vi "Debug C API.vi"() -> ()   [LabVIEW 2023]
doc: "Example to verify functionality using cAPIs"
panel:
  in  "CAPI Path":path
  in  "Output channel name":string[](array[string])=["Connector0_DIOPORT2", "Connector0_DIOPORT3", "Connector1_DIOPORT2", "Connector1_DIOPORT3"]
  in  "Channel data":u8[](array[numeric])=[255, 50, 100, 200]
  in  "Input channel names":string[](array[string])=["Connector0_DIOPORT0", "Connector0_DIOPORT1", "Connector1_DIOPORT0", "Connector1_DIOPORT1"]
  in  "Bit file name":string="RSeries7822R_ReadWriteDigitalPorts.lvbitx"
  in  "Resource":string="RIO_7822R_C1_S06"
  out "Channel data out":u8[](array[numeric])
  out "error out":errorcluster
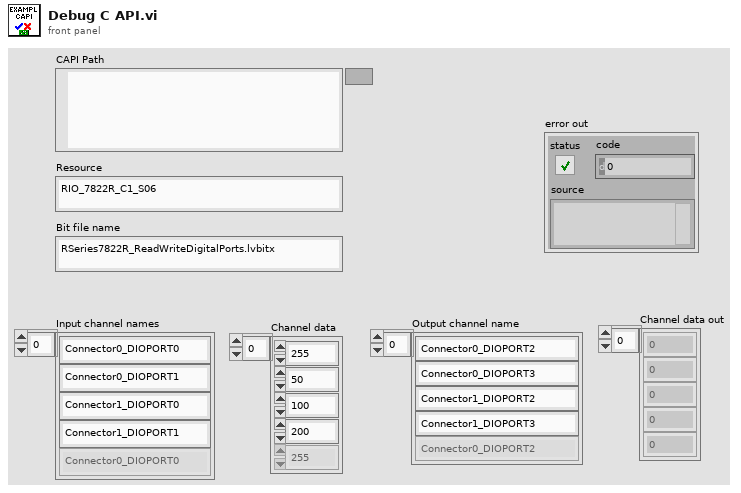
[diagram p1: front panel]
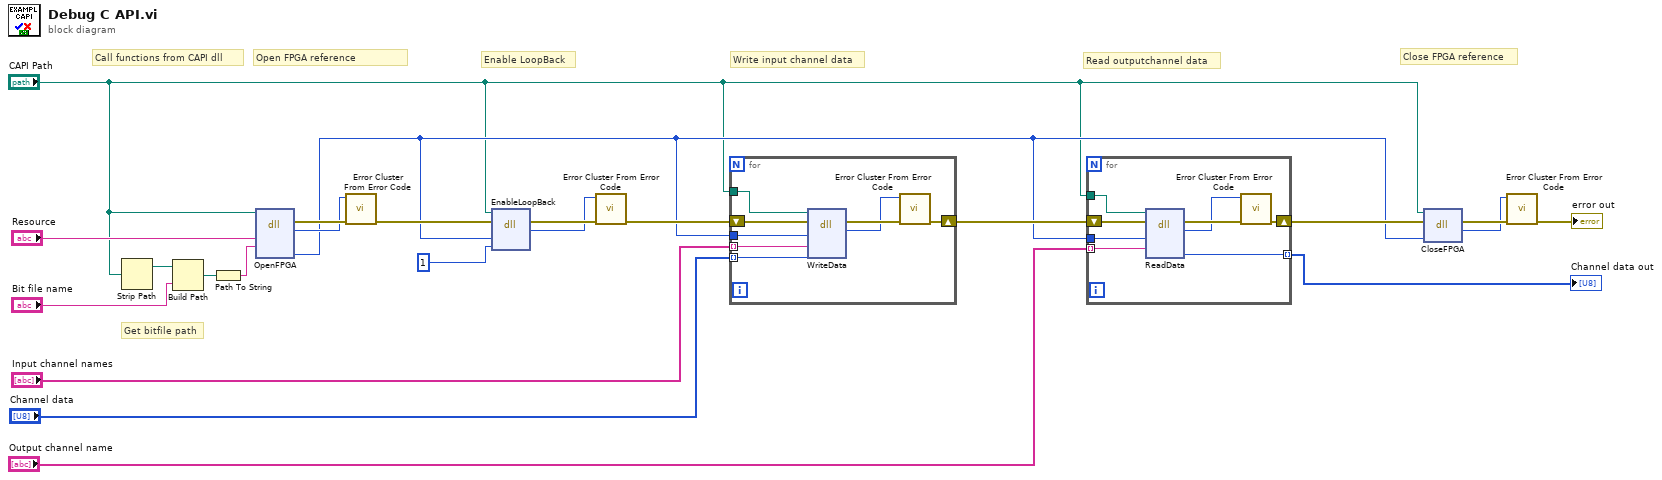
[diagram p0: block diagram]
diagram:
  # "Get bitfile path"
  # "Close FPGA reference"
  # "Read outputchannel data"
  # "Write input channel data"
  # "Enable LoopBack"
  # "Open FPGA reference"
  # "Call functions from CAPI dll"
  n1 = Strip Path(path="CAPI Path") -> (stripped path=w3:path)  [unwired: 1 out]
  n2 = Build Path(base path=w3, name or relative path="Bit file name") -> (appended path=w1:path)
  n3 = Path To String(path=w1) -> (string=w22:string)
  n4 = dll-call lib="C:/Users/Administrator/Desktop/RSeriesExample/Code Modules/Imports/RSeries7822RDriverAPI/RSeries7822R_ReadWriteDigitalPorts_CAPI.dll" fn="OpenFPGA"(path in="CAPI Path", "Resource"="Resource", "BitFile"=w22) -> (error out=w12:errorcluster, "return type"=w8:i32, "ReferenceOut"=w6:u64)  [unwired: 5 in, 1 out]
  n5 = call <vilib>:"Error Cluster From Error Code.vi"("error in (no error)"=w12, "error code (0)"=w8) -> ("error out"=w11:errorcluster)  [unwired: 7 in]
  n6 = dll-call lib="C:/Users/Administrator/Desktop/RSeriesExample/Code Modules/Imports/RSeries7822RDriverAPI/RSeries7822R_ReadWriteDigitalPorts_CAPI.dll" fn="EnableLoopBack"(path in="CAPI Path", error in=w11, "Reference"=w6, "EnableLoopBack"=u64 1) -> (error out=w20:errorcluster, "return type"=w7:i32)  [unwired: 3 in, 1 out]
  n7 = call <vilib>:"Error Cluster From Error Code.vi"("error in (no error)"=w20, "error code (0)"=w7) -> ("error out"=w10:errorcluster)  [unwired: 7 in]
  n8 = for {
    tunnel: w6 -> [w31]
    tunnel: "Input channel names" -> [w29] mode=indexing
    tunnel: "Channel data" -> [w30] mode=indexing
    shift-right: [w25] -> w19
    shift-left: w10 -> [w28]
    tunnel: "CAPI Path" -> [w26]
    n9 = dll-call lib="C:/Users/Administrator/Desktop/RSeriesExample/Code Modules/Imports/RSeries7822RDriverAPI/RSeries7822R_ReadWriteDigitalPorts_CAPI.dll" fn="WriteData"(path in=w26, error in=w28, "Reference"=w31, "ChannelName"=w29, "Data"=w30) -> (error out=w27:errorcluster, "return type"=w24:i32)  [unwired: 4 in, 1 out]
    n10 = call <vilib>:"Error Cluster From Error Code.vi"("error in (no error)"=w27, "error code (0)"=w24) -> ("error out"=w25:errorcluster)  [unwired: 7 in]
  }
  n11 = for {
    tunnel: w6 -> [w39]
    tunnel: "Output channel name" -> [w38] mode=indexing
    tunnel: [w37] -> w13 mode=indexing
    shift-right: [w33] -> w21
    shift-left: w19 -> [w36]
    tunnel: "CAPI Path" -> [w34]
    n12 = dll-call lib="C:/Users/Administrator/Desktop/RSeriesExample/Code Modules/Imports/RSeries7822RDriverAPI/RSeries7822R_ReadWriteDigitalPorts_CAPI.dll" fn="ReadData"(path in=w34, error in=w36, "Reference"=w39, "ChannelName"=w38) -> (error out=w35:errorcluster, "return type"=w32:i32, "Data"=w37:u8)  [unwired: 4 in, 1 out]
    n13 = call <vilib>:"Error Cluster From Error Code.vi"("error in (no error)"=w35, "error code (0)"=w32) -> ("error out"=w33:errorcluster)  [unwired: 7 in]
  }
  "Channel data out" <- w13
  n14 = dll-call lib="C:/Users/Administrator/Desktop/RSeriesExample/Code Modules/Imports/RSeries7822RDriverAPI/RSeries7822R_ReadWriteDigitalPorts_CAPI.dll" fn="CloseFPGA"(path in="CAPI Path", error in=w21, "Reference"=w6) -> (error out=w18:errorcluster, "return type"=w5:i32)  [unwired: 2 in, 1 out]
  n15 = call <vilib>:"Error Cluster From Error Code.vi"("error in (no error)"=w18, "error code (0)"=w5) -> ("error out"=→"error out":errorcluster)  [unwired: 7 in]
